vi "Read Roles.vi"(8 "error in (no error)":errorcluster, 11 "PenaltyEnemyPlayVSS in":refnum<class "PenaltyEnemyPlayVSS.lvclass">) -> (0 "error out":errorcluster, 2 "Roles":T1, 3 "PenaltyEnemyPlayVSS out":refnum<class "PenaltyEnemyPlayVSS.lvclass">)   [LabVIEW 2023, in "PenaltyEnemyPlayVSS.lvclass"]
uses:
  PenaltyEnemyPlayVSS.lvclass
  KeeperRoleVSS_class/KeeperRoleVSS.lvclass
  HaltRole_class/HaltRole.lvclass
  PenaltyEnemyPlayVSS.lvclass/PenaltyEnemyPlayVSS.ctl
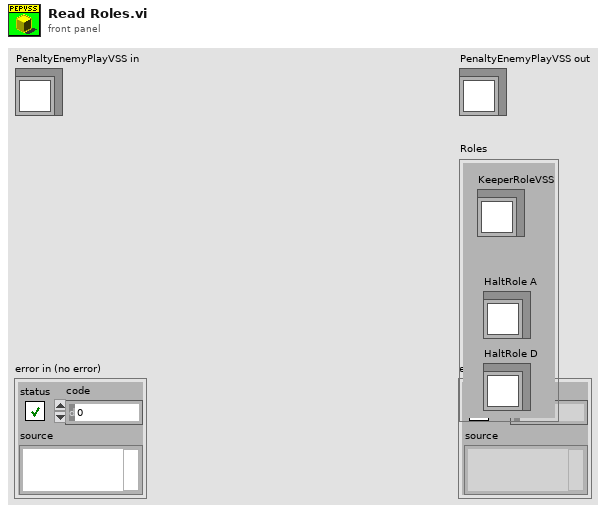
[diagram p1: front panel]
types:
  T1 = cluster{"KeeperRoleVSS":refnum<class "KeeperRoleVSS.lvclass">, "HaltRole A":refnum<class "HaltRole.lvclass">, "HaltRole D":refnum<class "HaltRole.lvclass">}
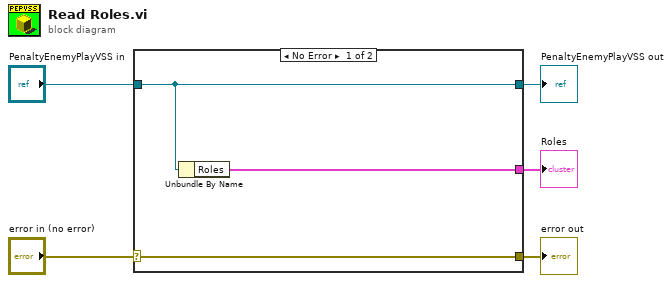
[diagram p0: block diagram]
diagram:
  n1 = case shown="No Error" "error in (no error)" {
    selector: "error in (no error)" -> [w8 w9]
    tunnel: [w8 w9] -> w4
    tunnel: [w7 w10] -> w2
    tunnel: "PenaltyEnemyPlayVSS in" -> [w7 w10]
    tunnel: [w6 _] -> w1
    frame No Error {
      n2 = Unbundle By Name(w7) -> ("Roles"=w6:T1)
    }
    frame Error {
    }
  }
  "error out" <- w4
  "PenaltyEnemyPlayVSS out" <- w2
  "Roles" <- w1
